vi "Set.vi"(6 "abort (F)":bool, 8 "element":T1={"Measurement type"=enum."Debug", "Sensor type"=enum."IFX_8in_256ch", "Identifier"="test.txt", "Open after execution?"=FALSE, "Plot after execution?"=FALSE, "Display channel"=0, "Voltage Delay (s)"=0.5, "Switch Delay (s)"=0.01, "VISA resource name source"="", "VISA resource name DMM"="", "VISA resource name LCR"="", "Compliance  Level (A)"=1e-05, "Voltage Limit (V)"=1000.0, "Data storage location"="", "Scan voltages"="", "Use source as DMM?"=FALSE, "LCR signal frequenzy (Hz)"=10000.0, "DMM device"=enum."Keithley2450", "Sampling number"=1, "Use env. sensors on"=enum."Sensirion sht1x/7x", "Switchboard Handle"=0, "Use Switchboard"=FALSE, "LCR signal voltage (V)"=10000.0, "Repeat"=1, "Scan voltages IV"="", "Scan voltages CV"="", "Hex pad numbers?"=FALSE, "Set measurement type"=enum."Debug", "Custom pad scan"="", "IV voltage Delay (s)"=0.5, "CV voltage Delay (s)"=0.5, "Needle measurement?"=FALSE, "Comments"="test.txt", "LCR signal frequenzy (kHz)"=10.0, "Compliance  Level (uA)"=10.0, "Open Correction Array"=array2304x3[6912 elements], "Current set voltage"=0.0, "Last set voltage"=0.0, "Current channel"=0, "Last OpenCorrection index"=-1, "Total curr/vltg every x steps"=10, "Current channel iteration"=0, "No CV corrections"=FALSE, "Mapfile"="", "Corrfile"="", "IV voltage file"=path "", "CV voltage file"=path "", "IV Switch Delay (s)"=0.01, "CV Switch Delay (s)"=0.01, "Invert polarity"=FALSE, "Set debug dirs"=FALSE, "Is n on p"=FALSE, "Source interlock?"=TRUE, "Voltage file used?"=FALSE, "Pad mask"="", "Mask pad above (uA)"=1.0, "LCR device"=enum."LCR_E4980", "Source device"=enum."Source_2410", "HexPlot binary path"=""} {"CV Switch Delay (s)" format="%#_13g"; "IV Switch Delay (s)" format="%#_13g"; "Last set voltage" format="%#_13g"; "Current set voltage" format="%#_13g"; "CV voltage Delay (s)" format="%#_13g"; "IV voltage Delay (s)" format="%#_13g"; "Voltage Limit (V)" format="%#_13g"; "Voltage Delay (s)" format="%#_13g"; "Switch Delay (s)" format="%#_13g"}, 11 "TagData in":refnum<class "TagData.lvclass">) -> (0 "previous element":T1={"Measurement type"=enum."Debug", "Sensor type"=enum."IFX_8in_256ch", "Identifier"="test.txt", "Open after execution?"=FALSE, "Plot after execution?"=FALSE, "Display channel"=0, "Voltage Delay (s)"=0.5, "Switch Delay (s)"=0.01, "VISA resource name source"="", "VISA resource name DMM"="", "VISA resource name LCR"="", "Compliance  Level (A)"=1e-05, "Voltage Limit (V)"=1000.0, "Data storage location"="", "Scan voltages"="", "Use source as DMM?"=FALSE, "LCR signal frequenzy (Hz)"=10000.0, "DMM device"=enum."Keithley2450", "Sampling number"=1, "Use env. sensors on"=enum."Sensirion sht1x/7x", "Switchboard Handle"=0, "Use Switchboard"=FALSE, "LCR signal voltage (V)"=10000.0, "Repeat"=1, "Scan voltages IV"="", "Scan voltages CV"="", "Hex pad numbers?"=FALSE, "Set measurement type"=enum."Debug", "Custom pad scan"="", "IV voltage Delay (s)"=0.5, "CV voltage Delay (s)"=0.5, "Needle measurement?"=FALSE, "Comments"="test.txt", "LCR signal frequenzy (kHz)"=10.0, "Compliance  Level (uA)"=10.0, "Open Correction Array"=array2304x3[6912 elements], "Current set voltage"=0.0, "Last set voltage"=0.0, "Current channel"=0, "Last OpenCorrection index"=-1, "Total curr/vltg every x steps"=10, "Current channel iteration"=0, "No CV corrections"=FALSE, "Mapfile"="", "Corrfile"="", "IV voltage file"=path "", "CV voltage file"=path "", "IV Switch Delay (s)"=0.01, "CV Switch Delay (s)"=0.01, "Invert polarity"=FALSE, "Set debug dirs"=FALSE, "Is n on p"=FALSE, "Source interlock?"=TRUE, "Voltage file used?"=FALSE, "Pad mask"="", "Mask pad above (uA)"=1.0, "LCR device"=enum."LCR_E4980", "Source device"=enum."Source_2410", "HexPlot binary path"=""} {"CV Switch Delay (s)" format="%#_13g"; "IV Switch Delay (s)" format="%#_13g"; "Last set voltage" format="%#_13g"; "Current set voltage" format="%#_13g"; "CV voltage Delay (s)" format="%#_13g"; "IV voltage Delay (s)" format="%#_13g"; "Voltage Limit (V)" format="%#_13g"; "Voltage Delay (s)" format="%#_13g"; "Switch Delay (s)" format="%#_13g"}, 1 "sequence":u64, 3 "TagData out":refnum<class "TagData.lvclass">, 4 "aborted?":bool)   [LabVIEW 2020, in "Tag-t'input_params.ctl'.lvlib" / "TagData.lvclass"]
uses:
  <extravilib>/ChannelInstances/Tag-t'input_params.ctl'/TagData.lvclass
  Desktop/HexDAQ/src/input_params.ctl
  <extravilib>/ChannelInstances/Tag-t'input_params.ctl'/TagData.lvclass/TagData.ctl
  <resource>/ChannelSupport/_ChannelSupport/_ChannelSupport.lvlib
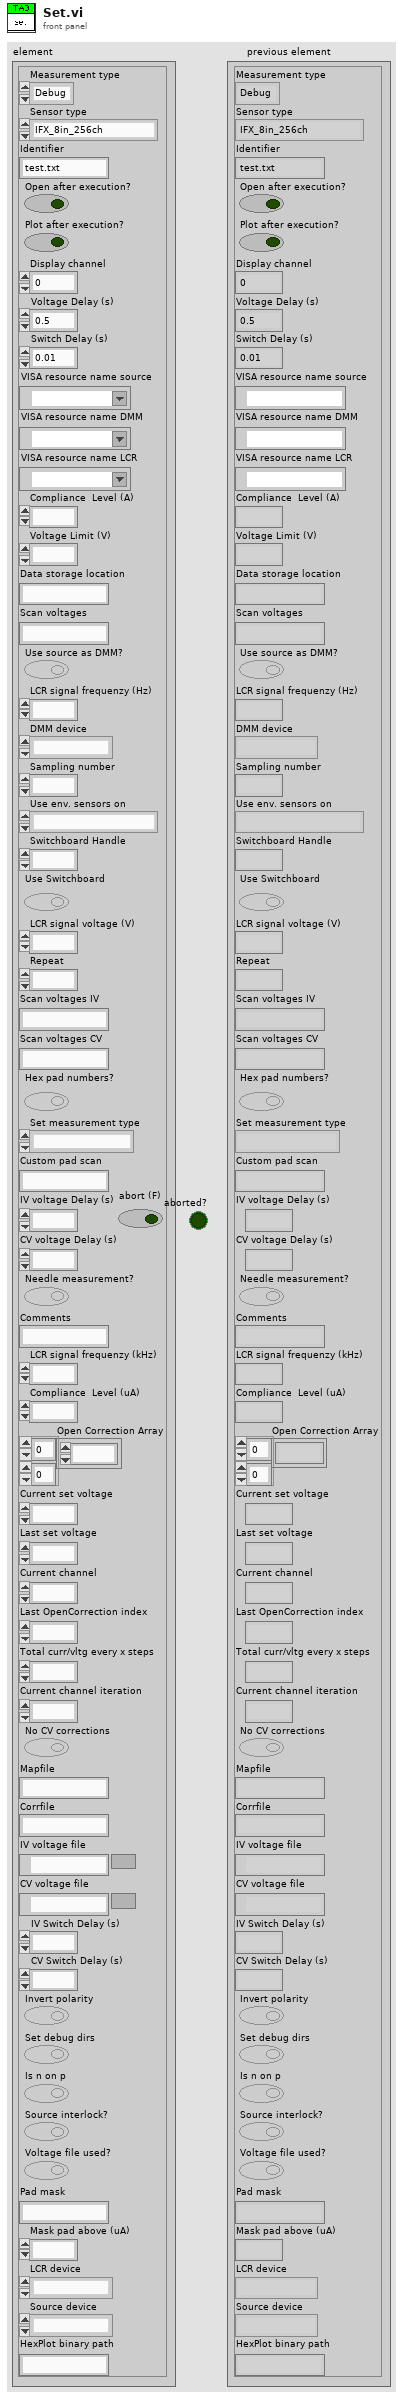
[diagram p1: front panel]
types:
  T1 = typedef "input_params.ctl" = cluster{"Measurement type":enum16{"IV", "CV", "Debug", "Test_contact"}, "Sensor type":enum16{"HPK_6in_135ch", "HPK_8in_271ch", "IFX_8in_256ch", "Diode", "HPK_6in_239ch", "Full_Matrix", "HPK_8in_271ch_full", "HPK_8in_198ch", "LumiCal", "HPK_8in_444ch", "HPK_8in_198ch_2019"}, "Identifier":string, "Open after execution?":bool, "Plot after execution?":bool, "Display channel":i32, "Voltage Delay (s)":dbl, "Switch Delay (s)":dbl, "VISA resource name source":refnum<visa-resource-name>, "VISA resource name DMM":refnum<visa-resource-name>, "VISA resource name LCR":refnum<visa-resource-name>, "Compliance  Level (A)":dbl, "Voltage Limit (V)":dbl, "Data storage location":string, "Scan voltages":string, "Use source as DMM?":bool, "LCR signal frequenzy (Hz)":dbl, "DMM device":enum16{"Keithley2001", "Keithley2450", "Keithley2410", "Keithley6485", "Keithley6487", "Keithley6517"}, "Sampling number":i32, "Use env. sensors on":enum16{"Sensirion sht1x/7x", "Switch Matrix", "Probecard"}, "Switchboard Handle":u32, "Use Switchboard":bool, "LCR signal voltage (V)":dbl, "Repeat":i32, "Scan voltages IV":string, "Scan voltages CV":string, "Hex pad numbers?":bool, "Set measurement type":enum16{"IV", "CV", "Debug", "Test_contact", "IV+CV"}, "Custom pad scan":string, "IV voltage Delay (s)":dbl, "CV voltage Delay (s)":dbl, "Needle measurement?":bool, "Comments":string, "LCR signal frequenzy (kHz)":dbl, "Compliance  Level (uA)":dbl, "Open Correction Array":dbl[][], "Current set voltage":dbl, "Last set voltage":dbl, "Current channel":i32, "Last OpenCorrection index":i32, "Total curr/vltg every x steps":i32, "Current channel iteration":i32, "No CV corrections":bool, "Mapfile":string, "Corrfile":string, "IV voltage file":path, "CV voltage file":path, "IV Switch Delay (s)":dbl, "CV Switch Delay (s)":dbl, "Invert polarity":bool, "Set debug dirs":bool, "Is n on p":bool, "Source interlock?":bool, "Voltage file used?":bool, "Pad mask":string, "Mask pad above (uA)":dbl, "LCR device":enum16{"LCR_E4980", "AGILENT_4263X"}, "Source device":enum16{"Source_2410", "Source_6487"}, "HexPlot binary path":string}
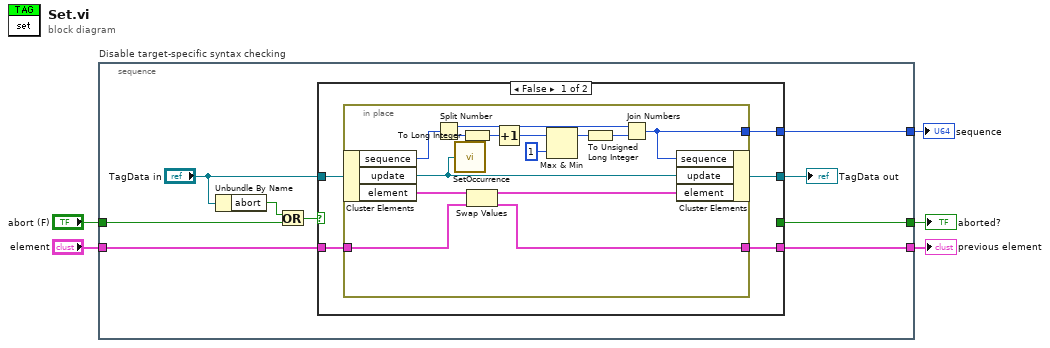
[diagram p0: block diagram]
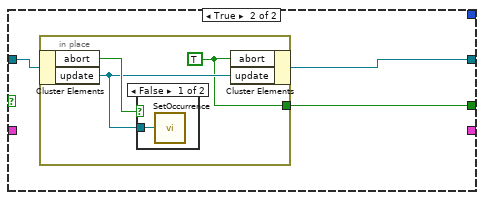
[diagram p2: hidden frame]
diagram:
  n1 = stacked-sequence "Disable target-specific syntax checking" {
    tunnel: "element" -> [w13]
    tunnel: [w12] -> w4
    tunnel: "abort (F)" -> [w9]
    tunnel: [w7] -> w2
    tunnel: [w6] -> w1
    frame #0 {
      n2 = Unbundle By Name("TagData in") -> ("abort"=w10:bool)
      n3 = Or(x=w10, y=w9) -> (x .or. y?=w8:bool)
      n4 = case shown="False" w8 {
        tunnel: [w19 w34] -> w14
        tunnel: w13 -> [w18 _]
        tunnel: [w17 _] -> w12
        tunnel: "TagData in" -> [w16 w36]
        tunnel: [_ w35] -> w7
        tunnel: [w15 _] -> w6
        frame False {
          n5 = in-place {
            in-place-border: w18 -> [w31]
            in-place-border: [w21] -> w17
            in-place-border: [w29] -> w15
            n6 = in-place-cluster #1(w16) -> ("sequence"=w22:u64, "update"=w30:refnum<k4>, "element"=w33:T1)
            n7 = Split Number(x=w22) -> (hi(x)=w23:u32, lo(x)=w27:u32)
            n8 = call <resource>:"SetOccurrence.vi"("occurrence"=w30) -> ()  [unwired: 9 in]
            n9 = To Long Integer(number=w27) -> (32bit integer=w25:i32)
            n10 = Swap Values(12:w33, 14:w31) -> (1:w32:T1, 3:w29:T1)  [unwired: 1 in]
            n11 = Increment(x=w25) -> (x+1=w28:i32)
            n12 = Max & Min(x=w28, y=1) -> (max(x,y)=w26:i32)  [unwired: 1 out]
            n13 = To Unsigned Long Integer(number=w26) -> (unsigned 32bit integer=w24:u32)
            n14 = Join Numbers(hi=w23, lo=w24) -> ((hi.lo)=w21:u64)
            n15 = in-place-cluster #1("sequence"=w21, "update"=w30, "element"=w32) -> (w19:refnum<class "TagData.lvclass">)
          }
        }
        frame True {
          n16 = in-place {
            in-place-border: [w37] -> w35
            w37 = TRUE ("abort")
            n17 = in-place-cluster #2(w36) -> ("abort"=w39:bool, "update"=w38:refnum<k4>)
            n18 = case shown="False" w39 {
              tunnel: w38 -> [w40 _]
              frame False {
                n19 = call <resource>:"SetOccurrence.vi"("occurrence"=w40) -> ()  [unwired: 9 in]
              }
              frame True {
              }
            }
            n20 = in-place-cluster #2("abort"=w37, "update"=w38) -> (w34:refnum<class "TagData.lvclass">)
          }
        }
      }
      "TagData out" <- w14
    }
  }
  "sequence" <- w4
  "aborted?" <- w2
  "previous element" <- w1
